vi "Air_Mass_Precess.vi"(0 "delta":dbl format="%07.9g", 3 "AH":dbl format="%07.9g") -> (6 "Air Mass":dbl)   [LabVIEW 2018]
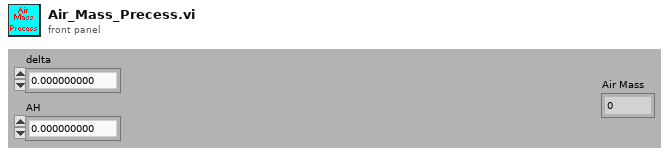
[diagram p1: front panel]
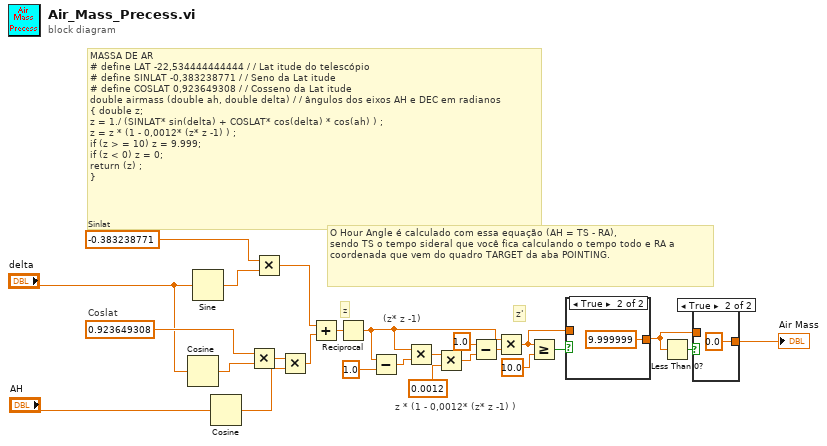
[diagram p0: block diagram]
diagram:
  # "z'"
  # "z * (1 - 0,0012* (z* z -1) )"
  # "(z* z -1)"
  # "z"
  # "O Hour Angle é calculado com essa equação (AH = TS - RA), \nsendo TS o tempo sideral que você fica calculando o tempo todo e RA a \ncoordenada que vem do quadro TARGET da aba POINTING."
  # "Coslat"
  # "Sinlat"
  # "MASSA DE AR\n# define LAT -22,534444444444 / / Lat itude do telescópio\n# define SINLAT -0,383238771 / / Seno da Lat itude\n# define COSLAT 0,923649308 / / Cosseno da Lat itude\ndouble airmass (double ah, double delta) / / ângulos dos eixos AH e DEC em radianos\n{ double z;\nz = 1./ (SINLAT* sin(delta) + COSLAT* cos(delta) * cos(ah) ) ;\nz = z * (1 - 0,0012* (z* z -1) ) ;\nif (z > = 10) z = 9.999;\nif (z < 0) z = 0;\nreturn (z) ;\n}"
  n1 = Cosine(x="delta") -> (cos(x)=w22:dbl)
  n2 = Sine(x="delta") -> (sin(x)=w24:dbl)
  n3 = Cosine(x="AH") -> (cos(x)=w20:dbl)
  n4 = Multiply(x=0.923649308 ("Delta=DEC"), y=w22) -> (x*y=w21:dbl)
  n5 = Multiply(x=-0.383238771 ("Delta=DEC"), y=w24) -> (x*y=w19:dbl)
  n6 = Multiply(x=w21, y=w20) -> (x*y=w18:dbl)
  n7 = Add(x=w19, y=w18) -> (x+y=w17:dbl)
  n8 = Reciprocal(x=w17) -> (1/x=w9:dbl)
  n9 = Subtract(x=w9, y=1.0) -> (x-y=w15:dbl)
  n10 = Multiply(x=w9, y=w15) -> (x*y=w14:dbl)
  n11 = Multiply(x=w14, y=0.0012) -> (x*y=w11:dbl)
  n12 = Subtract(x=1.0 ("y"), y=w11) -> (x-y=w10:dbl)
  n13 = Multiply(x=w9, y=w10) -> (x*y=w6:dbl)
  n14 = Greater Or Equal?(x=w6, y=10.0) -> (x >= y?=w7:bool)
  n15 = case shown="True" w7 {
    tunnel: [w26 9.999999 ("y")] -> w4
    tunnel: w6 -> [w26 _]
    frame False {
    }
    frame True {
    }
  }
  n16 = Less Than 0?(x=w4) -> (x < 0?=w5:bool)
  n17 = case shown="True" w5 {
    tunnel: [w28 0.0 ("y")] -> w3
    tunnel: w4 -> [w28 _]
    frame False {
    }
    frame True {
    }
  }
  "Air Mass" <- w3
